vi "Start_aquisition.vi"(8 "error in (no error)":errorcluster, 11 ".NET Refnum in":refnum<k24>) -> (0 "error out":errorcluster, 3 ".NET Refnum Out":refnum<k24>)   [LabVIEW 2021]
uses:
  C:/Program Files/Thorlabs/Scientific Imaging/ThorCam/uc480DotNet.dll
  Program Files/Thorlabs/Scientific Imaging/ThorCam/uc480DotNet.dll
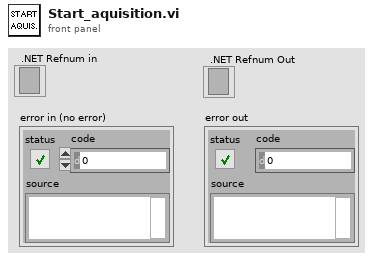
[diagram p1: front panel]
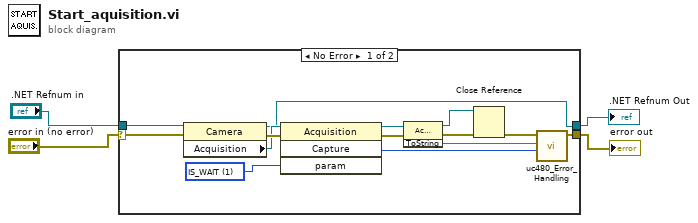
[diagram p0: block diagram]
diagram:
  n1 = case shown="No Error" "error in (no error)" {
    selector: "error in (no error)" -> [w7 w20]
    tunnel: [w13 w20] -> w4
    tunnel: ".NET Refnum in" -> [w6 w19]
    tunnel: [w5 w19] -> w1
    frame No Error {
      w15 = 1 items=["IS_DONT_WAIT", "IS_WAIT"] ("Wait")
      n2 = property class="Camera"(reference=w6, error in=w7) -> (reference out=w5:refnum<k24>, error out=w9:errorcluster, "Acquisition"=w8:refnum<k24>)
      n3 = invoke class="Acquisition" method="Capture"(reference=w8, error in=w9, "param"=w15) -> (reference out=w12:refnum<k24>, error out=w11:errorcluster, "Capture"=w14:i32)  [unwired: 1 in, 1 out]
      n4 = invoke class="Acquisition" method="ToString"(reference=w12, error in=w11) -> (reference out=w18:refnum<k24>, error out=w16:errorcluster, "ToString"=w10:string)  [unwired: 1 in]
      n5 = Close Reference(reference=w18, error in (no error)=w16) -> (error out=w17:errorcluster)
      n6 = call "uc480_Error_Handling.vi"("Error Code"=w14, "Error String"=w10, "Error In"=w17) -> ("Error Out"=w13:errorcluster)  [unwired: 8 in]
    }
    frame Error {
    }
  }
  "error out" <- w4
  ".NET Refnum Out" <- w1
